vi "ResetControlSub.vi"(0 "dt":dbl, 1 "Torque":bool, 2 "ResetAngle":dbl, 5 "TorqueSample0":dbl, 7 "Angel":bool, 9 "AngleSample0":dbl, 11 "ChannelStatus":T1 items=["通道关", "位置通道", "加载通道"], 12 "ResetTorque":dbl, 13 "ControlPara":dbl[](array[numeric])) -> (4 "ResetTorque 2":dbl, 6 "ResetAngle 2":dbl, 10 "ControlOutput":dbl, 15 "Commandout":dbl)   [LabVIEW 2011]
uses:
  Control 1.ctl
  <vilib>/addons/control/pid/pid.llb/PID (DBL).vi
  <vilib>/addons/control/pid/NI_PID_pid.lvlib
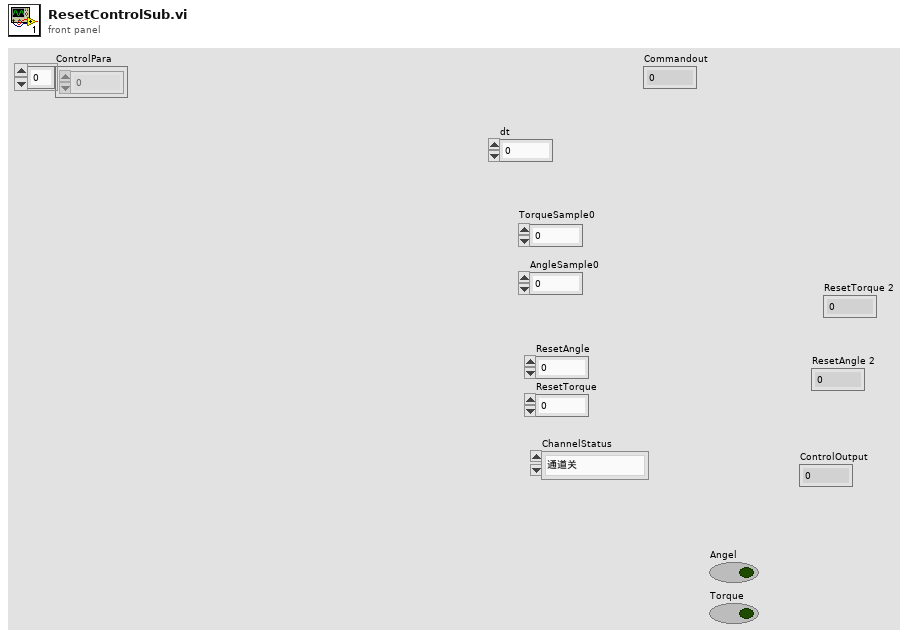
[diagram p1: front panel]
types:
  T1 = typedef "Control 1.ctl" = i32
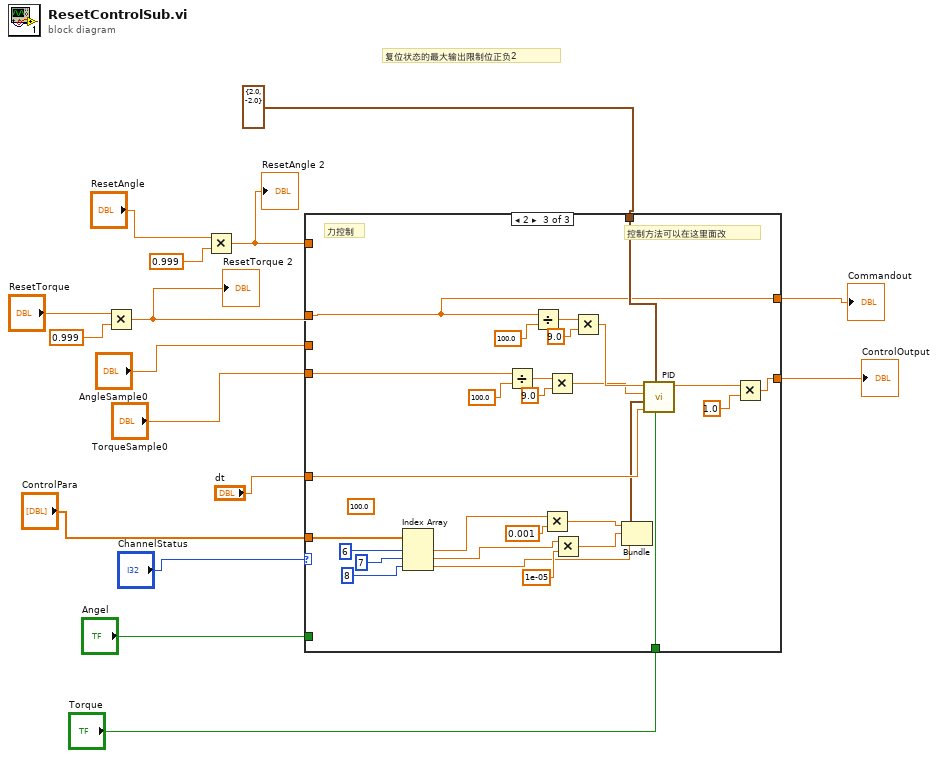
[diagram p0: block diagram]
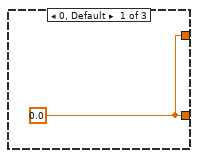
[diagram p2: hidden frame]
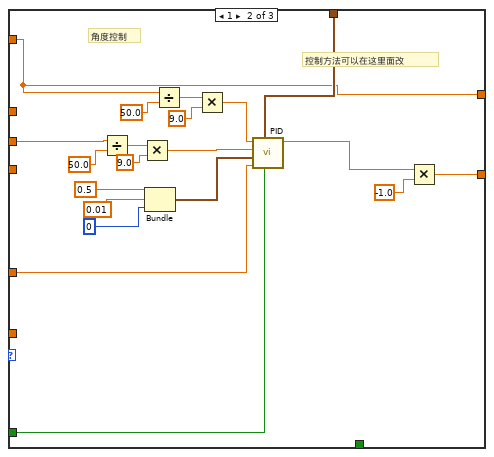
[diagram p3: hidden frame]
diagram:
  # "复位状态的最大输出限制位正负2"
  n1 = Multiply(x="ResetTorque", y=0.999) -> (x*y=w11:dbl)
  "ResetTorque 2" <- w11
  n2 = Multiply(x="ResetAngle", y=0.999) -> (x*y=w10:dbl)
  "ResetAngle 2" <- w10
  n3 = case shown="2" "ChannelStatus" {
    tunnel: "dt" -> [_ w37 w65]
    tunnel: [w17 w21 w53] -> w5
    tunnel: cluster{"output high":dbl, "output low":dbl} {"output high"=2.0, "output low"=-2.0} ("output range") -> [_ w36 w64]
    tunnel: w11 -> [_ _ w49]
    tunnel: w10 -> [_ w18 _]
    tunnel: "TorqueSample0" -> [_ _ w51]
    tunnel: "AngleSample0" -> [_ w20 _]
    tunnel: "Angel" -> [_ w19 _]
    tunnel: "Torque" -> [_ _ w50]
    tunnel: [w17 w18 w49] -> w2
    tunnel: "ControlPara" -> [_ _ w38]
    frame 0, Default {
      w17 = 0.0 ("output")
    }
    frame 1 {
      # "控制方法可以在这里面改"
      # "角度控制"
      n4 = Divide(x=w20, y=50.0) -> (x/y=w32:dbl)
      n5 = Multiply(x=w32, y=9.0) -> (x*y=w31:dbl)
      n6 = Bundle(0.5, 0.01, 0) -> (w35:cluster{dbl, dbl, i32})  [unwired: 1 in]
      n7 = Divide(x=w18, y=50.0) -> (x/y=w28:dbl)
      n8 = Multiply(x=w28, y=9.0) -> (x*y=w27:dbl)
      n9 = call-poly <vilib>:"PID.vi"("reinitialize? (F)"=w19, "output range"=w36, "dt (s)"=w37, "PID gains"=w35, "process variable"=w31, "setpoint"=w27) -> ("output"=w25:dbl)  [unwired: 4 in, 1 out]
      n10 = Multiply(x=w25, y=-1.0) -> (x*y=w21:dbl)
    }
    frame 2 {
      (unwired) 100.0 ("y")
      # "力控制"
      # "控制方法可以在这里面改"
      n11 = Index Array(array=w38, index #1=6 ("index"), index #2=7 ("index"), index #3=8 ("index")) -> (element #1=w42:dbl, element #2=w43:dbl, element #3=w39:dbl)
      n12 = Divide(x=w51, y=100.0) -> (x/y=w57:dbl)
      n13 = Divide(x=w49, y=100.0) -> (x/y=w61:dbl)
      n14 = Multiply(x=w42, y=0.001) -> (x*y=w41:dbl)
      n15 = Multiply(x=w57, y=9.0) -> (x*y=w56:dbl)
      n16 = Multiply(x=w43, y=1e-05) -> (x*y=w40:dbl)
      n17 = Multiply(x=w61, y=9.0) -> (x*y=w60:dbl)
      n18 = Bundle(w41, w40, "Numeric"=w39) -> (w54:cluster{dbl, dbl, "Numeric":dbl})  [unwired: 1 in]
      n19 = call-poly <vilib>:"PID.vi"("reinitialize? (F)"=w50, "output range"=w64, "dt (s)"=w65, "PID gains"=w54, "process variable"=w56, "setpoint"=w60) -> ("output"=w52:dbl)  [unwired: 4 in, 1 out]
      n20 = Multiply(x=w52, y=1.0) -> (x*y=w53:dbl)
    }
  }
  "ControlOutput" <- w5
  "Commandout" <- w2
